vi "Discrete Filter (DBL).vi"(2 "initialize":bool, 3 "filter coefficients":T1 {"reverse coefficients" format="%.2f"; "forward coefficients" format="%.2f"}, 5 "input data":dbl format="%.2f") -> (1 "output data":dbl format="%.2f")   [LabVIEW 2017, in "NI_AdvCtrl_discrete linear.lvlib"]
doc: "LabVIEW no longer supports this VI. You can obtain similar functionality by installing the LabVIEW Simulation Module.\n\nFilters the set of input data using the direct form IIR filter specified by Reverse Coefficients and Forward Coefficients."
uses:
  <vilib>/addons/control/advanced/NI_AdvCtrl_discrete linear.lvlib
  <vilib>/addons/control/advanced/NI_AdvCtrl_continuous linear.lvlib
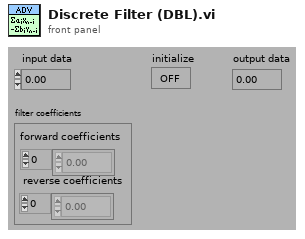
[diagram p1: front panel]
types:
  T1 = cluster{"forward coefficients":dbl[], "reverse coefficients":dbl[]}
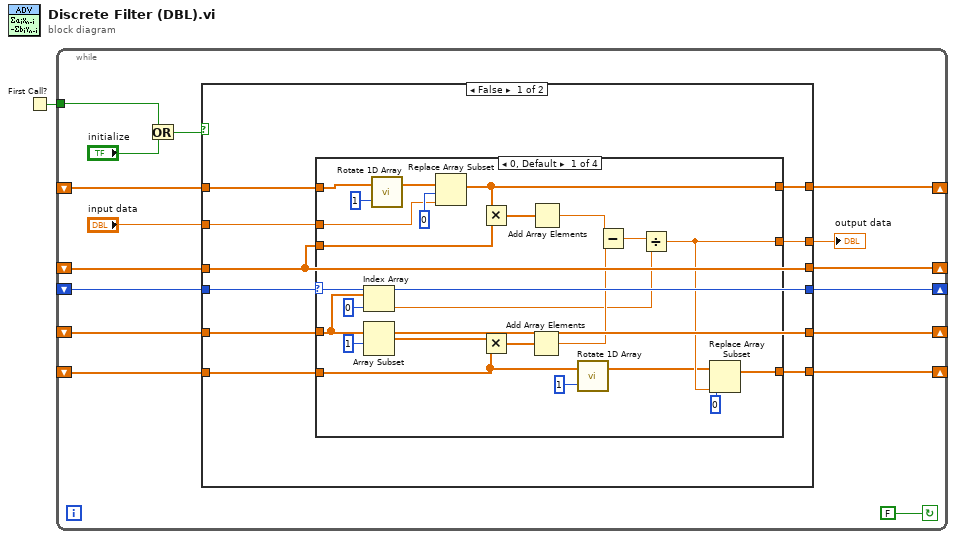
[diagram p0: block diagram]
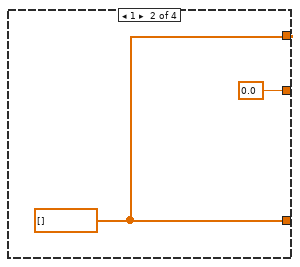
[diagram p2: hidden frame]
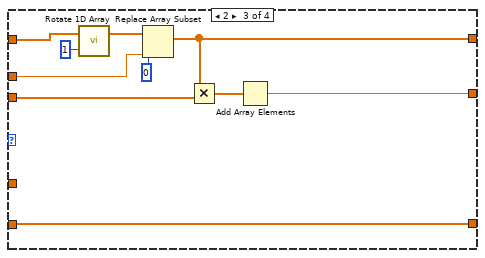
[diagram p3: hidden frame]
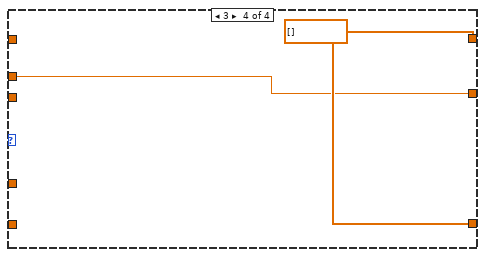
[diagram p4: hidden frame]
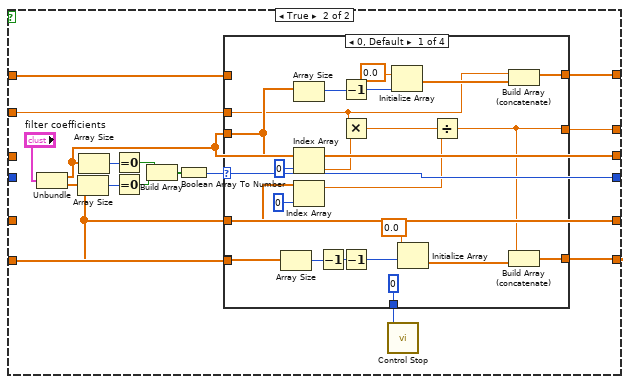
[diagram p5: hidden frame]
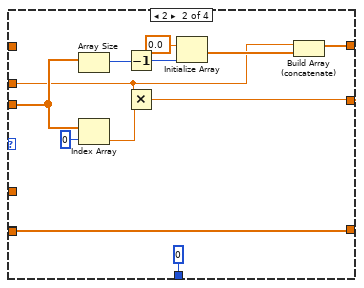
[diagram p6: hidden frame]
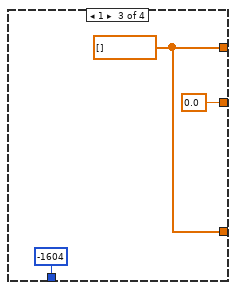
[diagram p7: hidden frame]
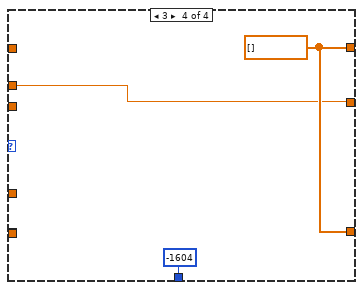
[diagram p8: hidden frame]
diagram:
  n1 = First Call?() -> (First Call?: T/F=w1:bool)
  n2 = while {
    shift-left: _ -> [w2]
    shift-right: [w3] -> _
    shift-left: _ -> [w5]
    shift-right: [w6] -> _
    shift-left: _ -> [w7]
    shift-right: [w8] -> _
    shift-left: _ -> [w10]
    shift-right: [w15] -> _
    shift-left: _ -> [w9]
    shift-right: [w14] -> _
    tunnel: w1 -> [w13]
    stop <- FALSE continue-if-true
    n3 = Or(x=w13, y="initialize") -> (x .or. y?=w11:bool)
    n4 = case shown="False" w11 {
      tunnel: w7 -> [w20 _]
      tunnel: w5 -> [w19 _]
      tunnel: w10 -> [w26 w75]
      tunnel: w9 -> [w25 w74]
      tunnel: [w21 w79] -> w16
      tunnel: [w24 w77] -> w15
      tunnel: [w23 w78] -> w14
      tunnel: "input data" -> [w22 w76]
      tunnel: [w20 w66] -> w8
      tunnel: [w19 w67] -> w6
      tunnel: [w18 w65] -> w3
      tunnel: w2 -> [w18 _]
      frame False {
        n5 = case shown="0, Default" w18 {
          tunnel: w26 -> [w32 _ w53 _]
          tunnel: w20 -> [w35 _ _ _]
          tunnel: w25 -> [w27 _ w55 _]
          tunnel: w19 -> [w41 _ w58 _]
          tunnel: [w42 w51 w56 w63] -> w24
          tunnel: [w44 w51 w55 w63] -> w23
          tunnel: w22 -> [w40 _ w59 w62]
          tunnel: [w37 0.0 ("Input_X") w57 w62] -> w21
          frame 0, Default {
            n6 = Index Array(array=w35, index=0 ("Index")) -> (element=w33:dbl)
            n7 = Array Subset(array=w35, index=1 ("Array Index")) -> (w39:dbl[])  [unwired: 1 in]
            n8 = call <vilib>:"Rotate 1D Array.vi"("n"=1, "array"=w32) -> ("array (last n elements first)"=w31:dbl[])  [unwired: 1 out]
            n9 = Replace Array Subset(array=w31, new element=w40, index=0 ("Index")) -> (w42:dbl[])
            n10 = Multiply(x=w42, y=w41) -> (x*y=w49:dbl[])
            n11 = Multiply(x=w39, y=w27) -> (x*y=w48:dbl[])
            n12 = Add Array Elements(numeric array=w48) -> (sum=w46:dbl)
            n13 = Add Array Elements(numeric array=w49) -> (sum=w47:dbl)
            n14 = call <vilib>:"Rotate 1D Array.vi"("n"=1, "array"=w27) -> ("array (last n elements first)"=w28:dbl[])  [unwired: 1 out]
            n15 = Subtract(x=w47, y=w46) -> (x-y=w36:dbl)
            n16 = Divide(x=w36, y=w33) -> (x/y=w37:dbl)
            n17 = Replace Array Subset(array=w28, new element=w37, index=0 ("Index")) -> (w44:dbl[])
          }
          frame 1 {
            w51 = dbl[] []
          }
          frame 2 {
            n18 = call <vilib>:"Rotate 1D Array.vi"("n"=1, "array"=w53) -> ("array (last n elements first)"=w54:dbl[])  [unwired: 1 out]
            n19 = Replace Array Subset(array=w54, new element=w59, index=0 ("Index")) -> (w56:dbl[])
            n20 = Multiply(x=w56, y=w58) -> (x*y=w61:dbl[])
            n21 = Add Array Elements(numeric array=w61) -> (sum=w57:dbl)
          }
          frame 3 {
            w63 = dbl[] []
          }
        }
      }
      frame True {
        n22 = Unbundle("filter coefficients") -> ("forward coefficients"=w67:dbl[], "reverse coefficients"=w66:dbl[])
        n23 = Array Size(array=w66) -> (size(s)=w70:i32)
        n24 = Array Size(array=w67) -> (size(s)=w71:i32)
        n25 = Equal To 0?(x=w71) -> (x = 0?=w69:bool)
        n26 = Equal To 0?(x=w70) -> (x = 0?=w68:bool)
        n27 = Build Array(w69, w68) -> (w72:bool[])
        n28 = Boolean Array To Number(Boolean array=w72) -> (number=w65:u32)
        n29 = case shown="0, Default" w65 {
          tunnel: w75 -> [_ _ _ _]
          tunnel: w66 -> [w93 w103 _ _]
          tunnel: w74 -> [_ _ _ _]
          tunnel: w67 -> [w92 w108 _ _]
          tunnel: [w85 w104 0.0 w118] -> w79
          tunnel: [w89 w105 w116 w119] -> w77
          tunnel: [w88 w103 w116 w119] -> w78
          tunnel: w76 -> [w90 w106 _ w118]
          tunnel: w66 -> [w83 _ _ _]
          tunnel: [0 0 -1604 -1604] -> w64
          frame 0, Default {
            n30 = Array Size(array=w93) -> (size(s)=w96:i32)
            n31 = Array Size(array=w92) -> (size(s)=w101:i32)
            n32 = Index Array(array=w92, index=0 ("Index")) -> (element=w97:dbl)
            n33 = Index Array(array=w83, index=0 ("Index")) -> (element=w81:dbl)
            n34 = Decrement(x=w96) -> (x-1=w86:i32)
            n35 = Decrement(x=w101) -> (x-1=w100:i32)
            n36 = Multiply(x=w90, y=w97) -> (x*y=w84:dbl)
            n37 = Decrement(x=w86) -> (x-1=w95:i32)
            n38 = Initialize Array(0.0 ("Element Data"), w100) -> (w91:dbl[])
            n39 = Initialize Array(0.0 ("Element Data"), w95) -> (w87:dbl[])
            n40 = Divide(x=w84, y=w81) -> (x/y=w85:dbl)
            n41 = Build Array (concatenate)(w90, w91) -> (w89:dbl[])
            n42 = Build Array (concatenate)(w85, w87) -> (w88:dbl[])
          }
          frame 2 {
            n43 = Array Size(array=w108) -> (size(s)=w113:i32)
            n44 = Index Array(array=w108, index=0 ("Index")) -> (element=w109:dbl)
            n45 = Decrement(x=w113) -> (x-1=w112:i32)
            n46 = Multiply(x=w106, y=w109) -> (x*y=w104:dbl)
            n47 = Initialize Array(0.0 ("Element Data"), w112) -> (w107:dbl[])
            n48 = Build Array (concatenate)(w106, w107) -> (w105:dbl[])
          }
          frame 1 {
            w116 = dbl[] []
          }
          frame 3 {
            w119 = dbl[] []
          }
        }
        n49 = call <vilib>:"Control Stop.vi"("error"=w64) -> ()  [unwired: 2 out]
      }
    }
    "output data" <- w16
  }
